vi "Close References.vi"(8 "error in":errorcluster, 11 "Controls/Indicators\nReferences":T1) -> (0 "error out":errorcluster)   [LabVIEW 2020]
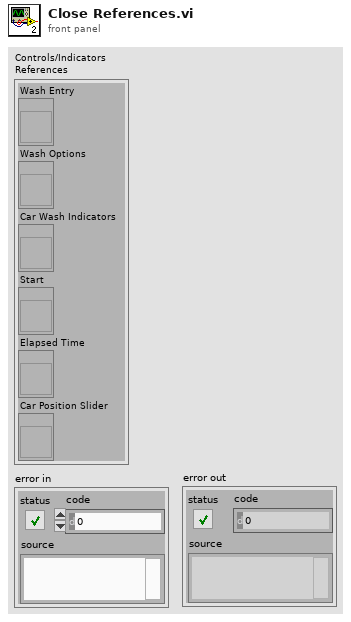
[diagram p1: front panel]
types:
  T1 = cluster{"Wash Entry":refnum<vi>, "Wash Options":refnum<vi>, "Car Wash Indicators":refnum<vi>, "Start":refnum<vi>, "Elapsed Time":refnum<vi>, "Car Position Slider":refnum<vi>}
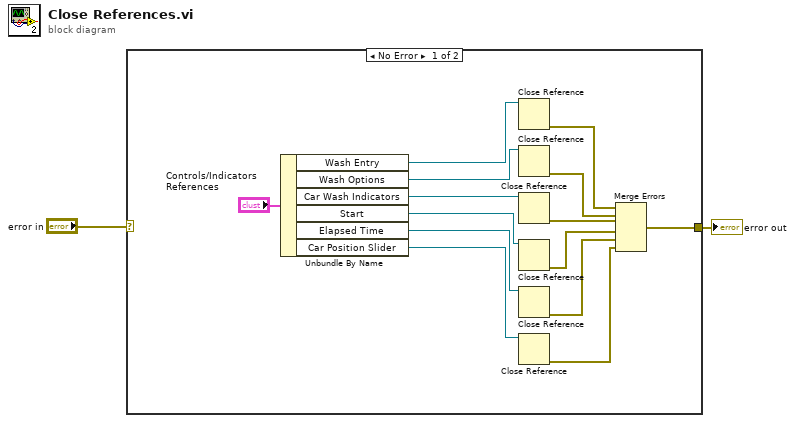
[diagram p0: block diagram]
diagram:
  n1 = case shown="No Error" "error in" {
    selector: "error in" -> [_ w17]
    tunnel: [w3 w17] -> w2
    frame No Error {
      n2 = Unbundle By Name("Controls/Indicators\nReferences") -> ("Wash Entry"=w16:refnum<vi>, "Wash Options"=w14:refnum<vi>, "Car Wash Indicators"=w13:refnum<vi>, "Start"=w10:refnum<vi>, "Elapsed Time"=w11:refnum<vi>, "Car Position Slider"=w12:refnum<vi>)
      n3 = Close Reference(reference=w16) -> (error out=w9:errorcluster)  [unwired: 1 in]
      n4 = Close Reference(reference=w14) -> (error out=w8:errorcluster)  [unwired: 1 in]
      n5 = Close Reference(reference=w13) -> (error out=w7:errorcluster)  [unwired: 1 in]
      n6 = Close Reference(reference=w10) -> (error out=w6:errorcluster)  [unwired: 1 in]
      n7 = Close Reference(reference=w11) -> (error out=w5:errorcluster)  [unwired: 1 in]
      n8 = Close Reference(reference=w12) -> (error out=w4:errorcluster)  [unwired: 1 in]
      n9 = Merge Errors(w9, w8, w7, w6, w5, w4) -> (w3:errorcluster)
    }
    frame Error {
    }
  }
  "error out" <- w2
